vi "Untitled 5.vi"() -> ()   [LabVIEW 2023]
uses:
  Glyph/Picture Control Canvas/Picture Control Canvas.lvclass
  Canvas/Drawer .Net.lvclass
  Glyph/Font Settings/Font Settings.lvclass
  LV-Awesome/LV Awesome/LV Awesome.lvclass
  E:/Labview/LV 2023/Libs/LV Symbol/LV Awesome/LV Awesome.lvclass
  E:/Labview/LV 2023/Libs/LV Symbol/Glyph/Glyph Source/Glyph Source.lvclass
  E:/Labview/LV 2023/Libs/LV Symbol/Glyph/Picture Control Canvas/Picture Control Canvas.lvclass
  E:/Labview/LV 2023/Libs/LV Symbol/Glyph/Glyph Canvas/Glyph Canvas.lvclass
panel:
  in  "Glyph Name":string="ei.blind"
  in  "Colors":T1={"Front"={"Color"=16711680, "Alpha"=255}, "Back"={"Color"=3381759, "Alpha"=255}}
  out "2D Picture":picture
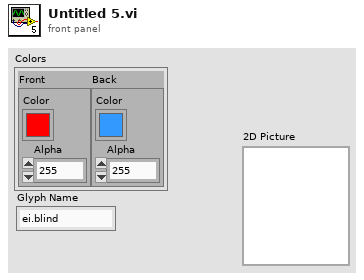
[diagram p1: front panel]
types:
  T1 = cluster{"Front":cluster{"Color":u32, "Alpha":u8}, "Back":cluster{"Color":u32, "Alpha":u8}}
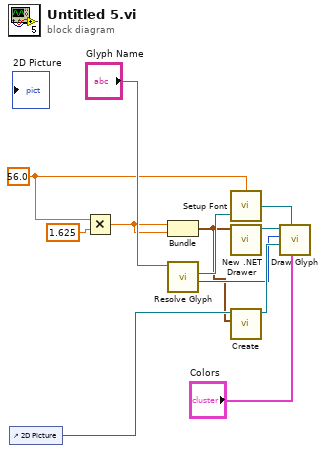
[diagram p0: block diagram]
diagram:
  w5 = 56.0 ("Size")
  n1 = control-ref of="2D Picture"() -> (w9:refnum<vi>)
  n2 = Multiply(x=w5, y=1.625) -> (x*y=w3:dbl)
  n3 = Bundle(w3, w3) -> (w2:cluster{dbl, dbl})  [unwired: 1 in]
  n4 = call-dynamic "Resolve Glyph.vi"("LV-Awesome.lvlib:LV Awesome.lvclass"="Glyph Name") -> ("charcode"=w6:u32, "Font Settings out"=w7:refnum<class "Font Settings.lvclass">)  [unwired: 7 in, 2 out]
  n5 = call "Setup Font.vi"("Size"=w5, "Font Path (System)"=w7) -> ("Font Settings out"=w12:refnum<class "Font Settings.lvclass">)  [unwired: 1 in]
  n6 = call "New .NET Drawer.vi"("Size"=w2) -> ("Canvas out"=w11:refnum<class "Drawer .Net.lvclass">)  [unwired: 9 in, 1 out]
  n7 = call "Create.vi"("Size (Full)"=w2, "2D Picture"=w9) -> ("Picture Control Canvas out"=w10:refnum<class "Picture Control Canvas.lvclass">)  [unwired: 8 in, 1 out]
  n8 = call-dynamic "Draw Glyph.vi"("Colors"="Colors", "Font (System)"=w12, "Destination"=w10, "codepoint"=w6, "Canvas .Net in"=w11) -> ()  [unwired: 4 in, 3 out]
